vi "Get LVClass Name from TD.vi"(8 "error in":errorcluster, 10 "Variant":variant) -> (0 "error out":errorcluster, 2 "LVClass Name":string)   [LabVIEW 2011, in "VITesterUtilities.lvlib"]
uses:
  Libraries/VITesterUtilities.lvlib
panel:
  out "value 2":u8
  out "value":u8
  out "Numeric":i32
  out "data string":string
  # "Copyright © 2007 James Kring, Inc. All rights reserved.\n\nAuthor: Jim Kring [jim.kring@jameskring.com]\n\nThis library is provided \"AS IS\" ,WITHOUT WARRANTIES OR \nCONDITIONS OF ANY KIND, either express or implied.\n\nJames Kring, Inc. -- http://www.jameskring.com"
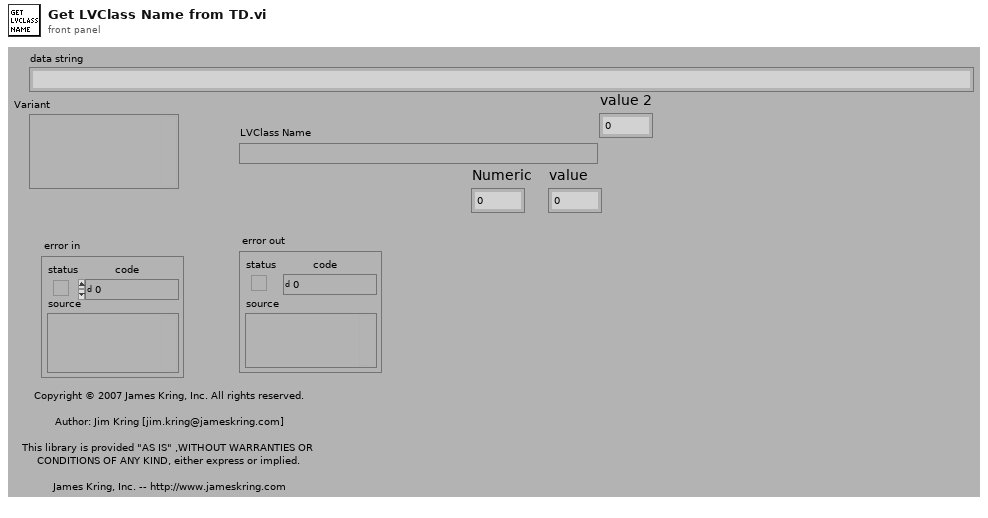
[diagram p1: front panel]
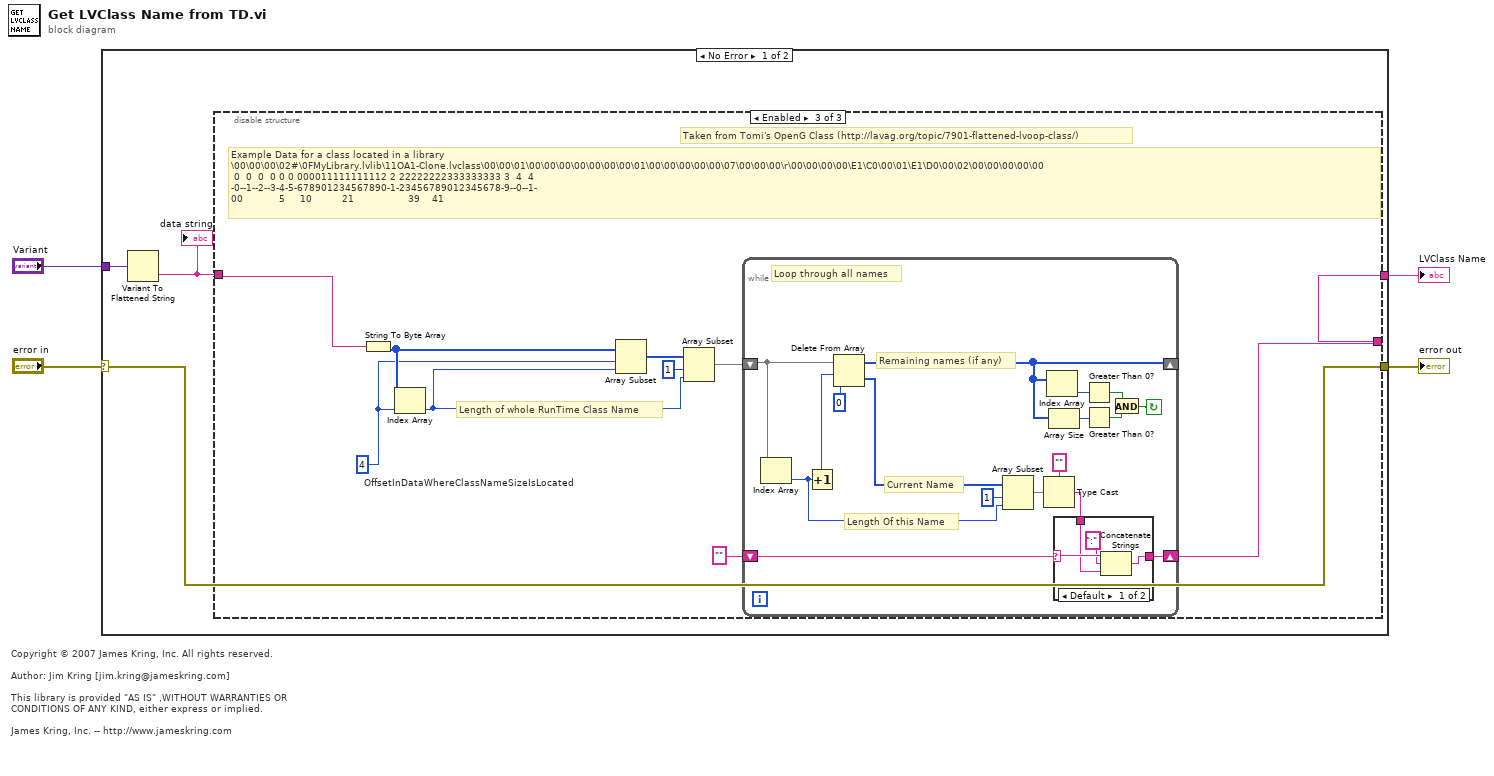
[diagram p0: block diagram]
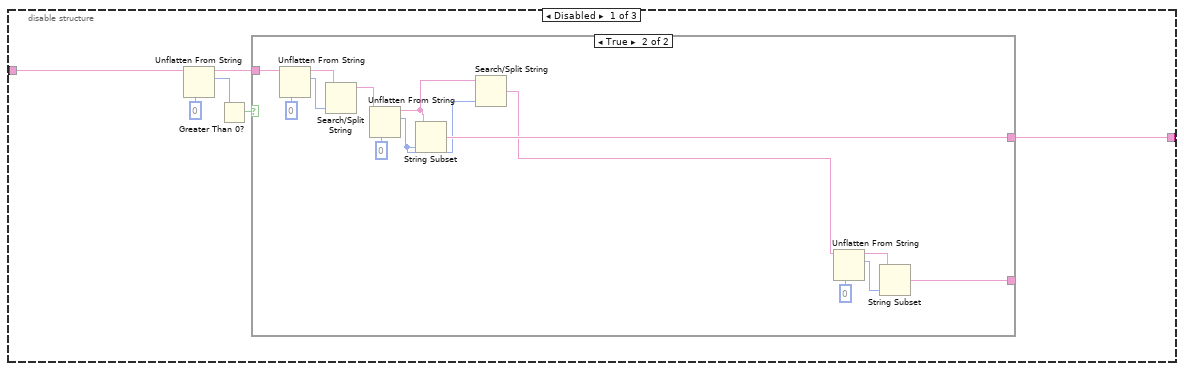
[diagram p2: hidden frame]
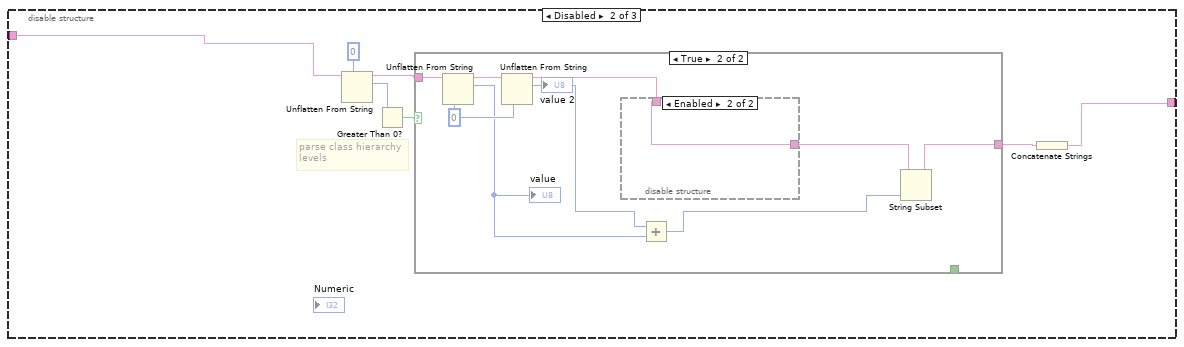
[diagram p4: hidden frame]
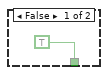
[diagram p5: hidden frame]
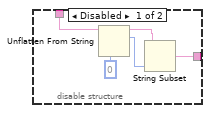
[diagram p6: hidden frame]
diagram:
  # "Copyright © 2007 James Kring, Inc. All rights reserved.\n\nAuthor: Jim Kring [jim.kring@jameskring.com]\n\nThis library is provided \"AS IS\" ,WITHOUT WARRANTIES OR \nCONDITIONS OF ANY KIND, either express or implied.\n\nJames Kring, Inc. -- http://www.jameskring.com"
  n1 = case shown="No Error" "error in" {
    selector: "error in" -> [w8 w83]
    tunnel: [w6 _] -> w4
    tunnel: "Variant" -> [w5 _]
    tunnel: [w8 w83] -> w1
    frame No Error {
      n2 = Variant To Flattened String(Variant=w5) -> (data string=w7:string)  [unwired: 1 out]
      "data string" <- w7
      n3 = disable-structure shown="Enabled" {
        disable-tunnel: w7 -> [w12 w35 w53]
        disable-tunnel: [w11 w33 w52] -> w6
        frame Disabled {
          n4 = Unflatten From String(type=u32 0, binary string=w12) -> (rest of the binary string=w13:string, value=w10:u32)  [unwired: 3 in, 1 out]
          n5 = Greater Than 0?(x=w10) -> (x > 0?=w9:bool)
          n6 = case shown="True" w9 {
            tunnel: w13 -> [_ w28]
            tunnel: [_ w27] -> w11
            tunnel: [_ w18] -> _
            frame False {
            }
            frame True {
              n7 = Unflatten From String(type=u8 0, binary string=w28) -> (rest of the binary string=w23:string, value=w24:u8)  [unwired: 3 in, 1 out]
              n8 = Search/Split String(string=w23, offset (0)=w24) -> (substring before match=w22:string)  [unwired: 1 in, 2 out]
              n9 = Unflatten From String(type=u8 0, binary string=w22) -> (rest of the binary string=w17:string, value=w16:u8)  [unwired: 3 in, 1 out]
              n10 = String Subset(string=w17, length (rest)=w16) -> (substring=w27:string)  [unwired: 1 in]
              n11 = Search/Split String(string=w17, offset (0)=w16) -> (match + rest of string=w15:string)  [unwired: 1 in, 2 out]
              n12 = Unflatten From String(type=u8 0, binary string=w15) -> (rest of the binary string=w19:string, value=w20:u8)  [unwired: 3 in, 1 out]
              n13 = String Subset(string=w19, length (rest)=w20) -> (substring=w18:string)  [unwired: 1 in]
            }
          }
        }
        frame Disabled {
          # "parse class hierarchy\nlevels"
          n14 = Unflatten From String(type=u32 0, binary string=w35) -> (rest of the binary string=w29:string, value=w31:u32)  [unwired: 3 in, 1 out]
          n15 = Greater Than 0?(x=w31) -> (x > 0?=w30:bool)
          n16 = case shown="True" w30 {
            tunnel: w29 -> [_ w45]
            tunnel: [_ w41] -> w34
            tunnel: [TRUE _] -> _
            frame False {
            }
            frame True {
              w43 = u8 0
              n17 = Unflatten From String(type=w43, binary string=w45) -> (rest of the binary string=w44:string, value=w39:u8)  [unwired: 3 in, 1 out]
              "value" <- w39
              n18 = Unflatten From String(type=w43, binary string=w44) -> (rest of the binary string=w42:string, value=w38:u8)  [unwired: 3 in, 1 out]
              "value 2" <- w38
              n19 = disable-structure shown="Enabled" {
                disable-tunnel: [w47 w51] -> w40
                disable-tunnel: w42 -> [w46 w51]
                frame Disabled {
                  n20 = Unflatten From String(type=u8 0, binary string=w46) -> (rest of the binary string=w49:string, value=w48:u8)  [unwired: 3 in, 1 out]
                  n21 = String Subset(string=w49, length (rest)=w48) -> (substring=w47:string)  [unwired: 1 in]
                }
                frame Enabled {
                }
              }
              n22 = Add(x=w38, y=w39) -> (x+y=w37:u8)
              n23 = String Subset(string=w40, length (rest)=w37) -> (substring=w41:string)  [unwired: 1 in]
            }
          }
          n24 = Concatenate Strings(w34) -> (w33:string)
        }
        frame Enabled {
          w57 = 4  # OffsetInDataWhereClassNameSizeIsLocated
          # "Taken from Tomi's OpenG Class (http://lavag.org/topic/7901-flattened-lvoop-class/)"
          # "Length of whole RunTime Class Name"
          # "Example Data for a class located in a library\n\\00\\00\\00\\02#\\0FMyLibrary.lvlib\\11OA1-Clone.lvclass\\00\\00\\01\\00\\00\\00\\00\\00\\00\\00\\01\\00\\00\\00\\00\\00\\07\\00\\00\\00\\r\\00\\00\\00\\00\\E1\\C0\\00\\01\\E1\\D0\\00\\02\\00\\00\\00\\00\\00\n 0  0  0  0 0 0 000011111111112 2 22222222333333333 3  4  4\n-0--1--2--3-4-5-678901234567890-1-23456789012345678-9--0--1-\n00            5     10          21                  39    41"
          n25 = String To Byte Array(string=w53) -> (unsigned byte array=w58:u8[])
          n26 = Index Array ("get len")(array=w58, index=w57) -> (element=w54:u8)
          n27 = Array Subset(array=w58, index=w57, length=w54) -> (w55:u8[])
          n28 = Array Subset(array=w55, index=1, length=w54) -> (w59:u8[])
          n29 = while {
            shift-right: [w66] -> _
            shift-left: w59 -> [w69]
            shift-right: [w71] -> w52
            shift-left: "" ("type") -> [w73]
            stop <- w62 continue-if-true
            # "Remaining names (if any)"
            # "Current Name"
            # "Loop through all names"
            # "Length Of this Name"
            n30 = Index Array ("get len")(array=w69) -> (element=w67:u8)  [unwired: 1 in]
            n31 = Increment(x=w67) -> (x+1=w68:u8)
            n32 = Delete From Array(array=w69, length=w68, index=0) -> (deleted portion=w61:u8[], array with subset deleted=w66:u8[])
            n33 = Array Subset(array=w61, index=1, length=w67) -> (w74:u8[])
            n34 = Type Cast(type="", x=w74) -> (*(type *) &x=w72:string)
            n35 = Index Array(array=w66) -> (element=w65:u8)  [unwired: 1 in]
            n36 = Array Size(array=w66) -> (size(s)=w70:i32)
            n37 = case shown="Default" w73 {
              selector: w73 -> [w81 _]
              tunnel: w72 -> [w79 w82]
              tunnel: [w78 w82] -> w71
              frame Default {
                n38 = Concatenate Strings(w81, ":" ("string"), w79) -> (w78:string)
              }
              frame "" {
              }
            }
            n39 = Greater Than 0?(x=w65) -> (x > 0?=w64:bool)
            n40 = Greater Than 0?(x=w70) -> (x > 0?=w63:bool)
            n41 = And(x=w64, y=w63) -> (x .and. y?=w62:bool)
          }
        }
      }
    }
    frame Error {
    }
  }
  "LVClass Name" <- w4
  "error out" <- w1
